vi "Build Wheel Speed Sensor Section.vi"(6 "Cancelled?":bool, 8 "error in (no error)":errorcluster, 9 "Card Position in":T1 {"Slot #" max=15}, 10 "Name in":string, 11 "Node Ptr in":u64) -> (0 "error out":errorcluster)   [LabVIEW 2014, in "SLSC configuration System Explorer.lvlib"]
uses:
  SLSC configuration System Explorer.lvlib
  Type Defs/Card Position.ctl
  Shared/SPI Utility/Slot #.ctl
  <vilib>/NI Veristand/Custom Device API/Custom Device Channel.ctl
  <vilib>/NI Veristand/Custom Device API/Custom Device Channel Type.ctl
  Shared/Constants.vi
  <vilib>/NI Veristand/Custom Device API/Set Item Property (U16).vi
  <vilib>/NI Veristand/Custom Device API/Custom Device API.lvlib
  Shared/SLSC configuration Shared.lvlib
  <vilib>/NI Veristand/Custom Device Tools/Custom Device Utility Library/Custom Device Utility Library.lvlib
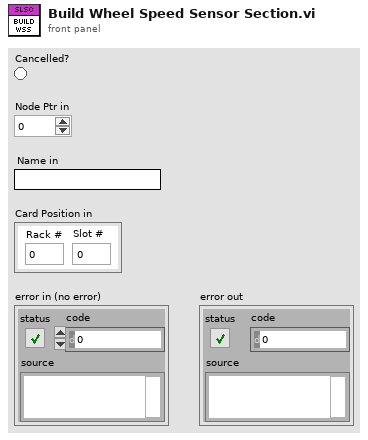
[diagram p1: front panel]
types:
  T1 = typedef "SLSC configuration Shared.lvlib/Card Position.ctl" = cluster{"Rack #":u8, "Slot #":T2}
  T2 = typedef "SLSC configuration Shared.lvlib/Slot #.ctl" = u8
  T3 = typedef "Custom Device API.lvlib/Custom Device Channel Type.ctl" = enum16{"Input", "Output"}
  T4 = typedef "Custom Device API.lvlib/Custom Device Channel.ctl" = cluster{"Type":T3, "Units":string, "Default Value":dbl, "Faultable":bool, "Scalable":bool}
  T5 = typedef "Custom Device API.lvlib/Custom Device Item Ref.ctl" = u64
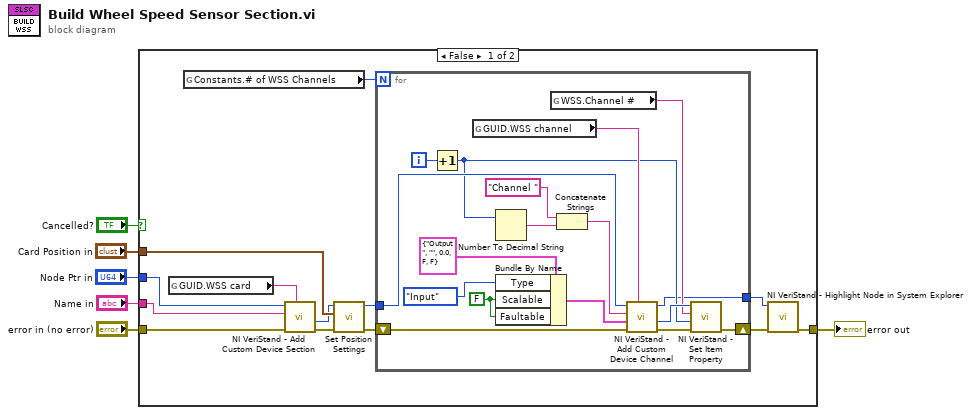
[diagram p0: block diagram]
diagram:
  n1 = case shown="False" "Cancelled?" {
    tunnel: "error in (no error)" -> [w19 w37]
    tunnel: "Node Ptr in" -> [w18 _]
    tunnel: "Card Position in" -> [w15 _]
    tunnel: [w8 w37] -> w5
    tunnel: "Name in" -> [w7 _]
    frame False {
      n2 = global read "Constants.vi" "GUID.WSS card"() -> (w17:string)
      n3 = global read "Constants.vi" "Constants.# of WSS Channels"() -> (w13:u8)
      n4 = call <vilib>:"NI VeriStand - Add Custom Device Section.vi"("GUID (Default Section)"=w17, "error in (no error)"=w19, "Section Name"=w7, "Parent Ref in"=w18) -> ("error out"=w16:errorcluster, "Section Ptr"=w14:T5)  [unwired: 4 in, 2 out]
      n5 = call "Set Position Settings.vi"("error in (no error)"=w16, "Card Position"=w15, "Item Ref in"=w14) -> ("error out"=w12:errorcluster, "Item Ref out"=w11:T5)  [unwired: 7 in]
      n6 = for {
        N: w13 -> [_]
        shift-right: [w21] -> w10
        shift-left: w12 -> [w32]
        tunnel: w11 -> [w25]
        tunnel: [w20] -> w9
        i -> [w31]
        w33 = FALSE ("Scalable")
        n7 = Increment(x=w31) -> (x+1=w22:i32)
        n8 = global read "Constants.vi" "GUID.WSS channel"() -> (w27:string)
        n9 = Number To Decimal String(number=w22) -> (decimal integer string=w30:string)  [unwired: 1 in]
        n10 = Bundle By Name(cluster=T4 {"Type"=enum."Output", "Units"="", "Default Value"=0.0, "Faultable"=FALSE, "Scalable"=FALSE} ("Channel"), "Type"=Custom_Device_Channel_Type."Input", "Scalable"=w33, "Faultable"=w33) -> (w35:T4)
        n11 = global read "Constants.vi" "WSS.Channel #"() -> (w23:string)
        n12 = Concatenate Strings("Channel " ("Channel Name"), w30) -> (w28:string)
        n13 = call <vilib>:"NI VeriStand - Add Custom Device Channel.vi"("GUID (Default Channel)"=w27, "error in (no error)"=w32, "Channel"=w35, "Channel Name"=w28, "Parent Ref in"=w25) -> ("error out"=w26:errorcluster, "Channel Ref"=w24:T5, "Parent Ref out"=w20:T5)  [unwired: 3 in, 1 out]
        n14 = call-poly <vilib>:"NI VeriStand - Set Item Property.vi"("error in (no error)"=w26, "Value"=w22, "Property Name"=w23, "Item Ref in"=w24) -> ("error out"=w21:errorcluster)  [unwired: 5 in, 2 out]
      }
      n15 = call <vilib>:"NI VeriStand - Highlight Node in System Explorer.vi"("error in (no error)"=w10, "Item Ref in"=w9) -> ("error out"=w8:errorcluster)  [unwired: 8 in, 1 out]
    }
    frame True {
    }
  }
  "error out" <- w5
